vi "Intake_Joint_Execute.vi"() -> ()   [LabVIEW 2018]
uses:
  <vilib>/Rock Robotics/WPI/DriverStation/WPI_DriverStationRobotMode2.ctl
  <vilib>/Rock Robotics/WPI/ThirdParty/Phoenix-LabVIEW/Motor Controller/Controls/CTRE_Phoenix_MotorControl_ControlMode.ctl
  Global_Variables/Intake_Joint_Globals.vi
  Global_Variables/Sensor_Values.vi
  Global_Variables/Robot_Global_Data.vi
  Global_Variables/Dashboard_Globals.vi
panel:
  in  "Current_Position":dbl
  in  "Max_Speed":dbl=0.75 format="%#_13g"
  in  "Gain_Down":dbl=0.00025
  in  "Gain_Up":dbl=0.0006
  in  "Decrement":dbl=60.0
  in  "Increment":dbl=60.0
  in  "Gain":dbl=0.0009
  in  "Down_Speed":dbl=-0.3
  in  "Up_Speed":dbl=0.35
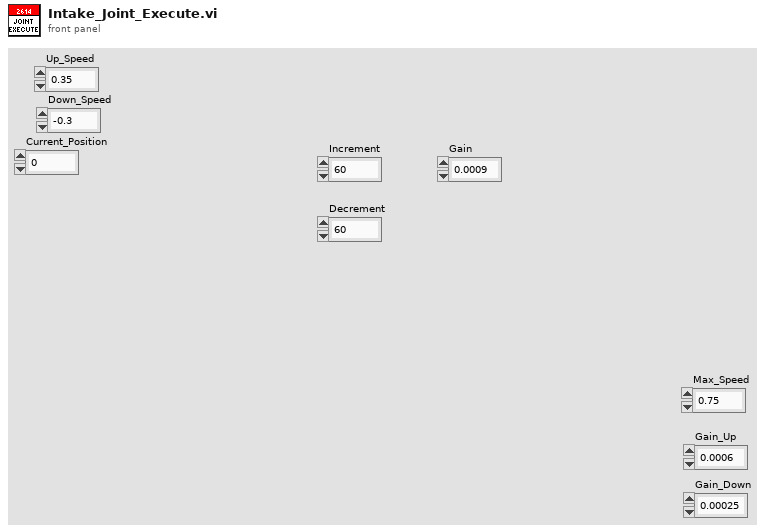
[diagram p1: front panel]
types:
  T1 = typedef "WPI_MotorControlDeviceRef.ctl" = cluster{"DeviceStatus":errorcluster, "Type":T2, "PWM":cluster{"PWM Channel":T3, "DeadBand":T4}, "CAN":cluster{"Device Number":u8, "SetOutput VI Ref":variant, "GetOutput VI Ref":variant, "Enable VI Ref":variant, "Disable VI Ref":variant, "Data":variant}, "Invert":bool, "DIO PWM":cluster{"PWM \"Enable\" Channel":T3, "DIOChannel":T5, "PWM Rate":dbl}}
  T2 = typedef "WPI_MotorControlType.ctl" = enum16{"PWM", "CAN", "DIO PWM"}
  T3 = typedef "FPGA_DIOPWMChannel.ctl" = enum8{"PWM 0", "PWM 1", "PWM 2", "PWM 3", "PWM 4", "PWM 5", "PWM 6", "PWM 7", "PWM 8", "PWM 9", "PWM MXP 0", "PWM MXP 1", "PWM MXP 2", "PWM MXP 3", "PWM MXP 4", "PWM MXP 5", "PWM MXP 6", "PWM MXP 7", "PWM MXP 8", "PWM MXP 9", "Invalid"}
  T4 = typedef "WPI_PWMDeadband.ctl" = cluster{"Name":string, "maxPositivePwm":i32, "minPositivePwm":i32, "centerPwm":i32, "maxNegativePwm":i32, "minNegativePwm":i32, "angularRange":u16}
  T5 = typedef "FPGA_DIOChannel.ctl" = enum8{"DIO 0", "DIO 1", "DIO 2", "DIO 3", "DIO 4", "DIO 5", "DIO 6", "DIO 7", "DIO 8", "DIO 9", "DIO MXP 0", "DIO MXP 1", "DIO MXP 2", "DIO MXP 3", "DIO MXP 4", "DIO MXP 5", "DIO MXP 6", "DIO MXP 7", "DIO MXP 8", "DIO MXP 9", "DIO MXP 10", "DIO MXP 11", "DIO MXP 12", "DIO MXP 13", "DIO MXP 14", "DIO MXP 15", "SPI Port CS1", "SPI Port CS2", "SPI Port CS3", "SPI Port MISO", "SPI Port MOSI", "Invalid"}
  T6 = typedef "WPI_DriverStationRobotMode2.ctl" = enum16{"Autonomous Disabled", "Autonomous Enabled", "Teleop Disabled", "Teleop Enabled", "Disconnected", "Finish", "Test Disabled", "Test Enabled", "Emergency Stopped"}
  T7 = typedef "Intake_Joint_Notifier.ctl" = cluster{"Intake_Joint_Control_Type":T8, "Manual_Joint_Up":bool, "Manual_Joint_Down":bool, "Low_Rocket":bool, "Mid_Rocket":bool, "High_Rocket":bool, "Cargo_Ship":bool, "Hatch_Floor":bool, "Cargo_Floor":bool, "HP_Hatch":bool, "HP_Cargo":bool, "Depot_Cargo":bool, "Stow":bool, "Intake_Mode":bool, "Set Position":T9, "Parameter_One":dbl, "Parameter_Two":dbl, "Parameter_Three":dbl, "Step":i32, "Joint_Notifier":refnum<notifier>}
  T8 = typedef "Intake_Joint_Control_Type.ctl" = enum16{"No_Op", "Manual_Joint_Up", "Manual_Joint_Down", "Manual_Position_Control", "Position_Control", "Position"}
  T9 = typedef "Intake_Joint_Enum_States.ctl" = enum16{"Current_Position", "High_Rocket_Hatch_Panel_Floor", "High_Rocket_Hatch_Panel", "Mid_Rocket_Hatch_Panel_Floor", "Mid_Rocket_Hatch_Panel", "Low_Rocket_Hatch_Panel", "Cargo_Ship_Hatch_Panel", "Loading_Station_Hatch_Panel", "Ground_Pickup_Hatch_Panel", "High_Rocket_Cargo", "Mid_Rocket_Cargo", "Low_Rocket_Cargo", "Cargo_Ship_Cargo", "Loading_Station_Cargo", "Ground_Pickup_Cargo", "Depot_Pickup_Cargo", "Stow_Cargo", "Get_Hatch"}
  T10 = typedef "CTRE_Phoenix_MotorControl_ControlMode.ctl" = u16
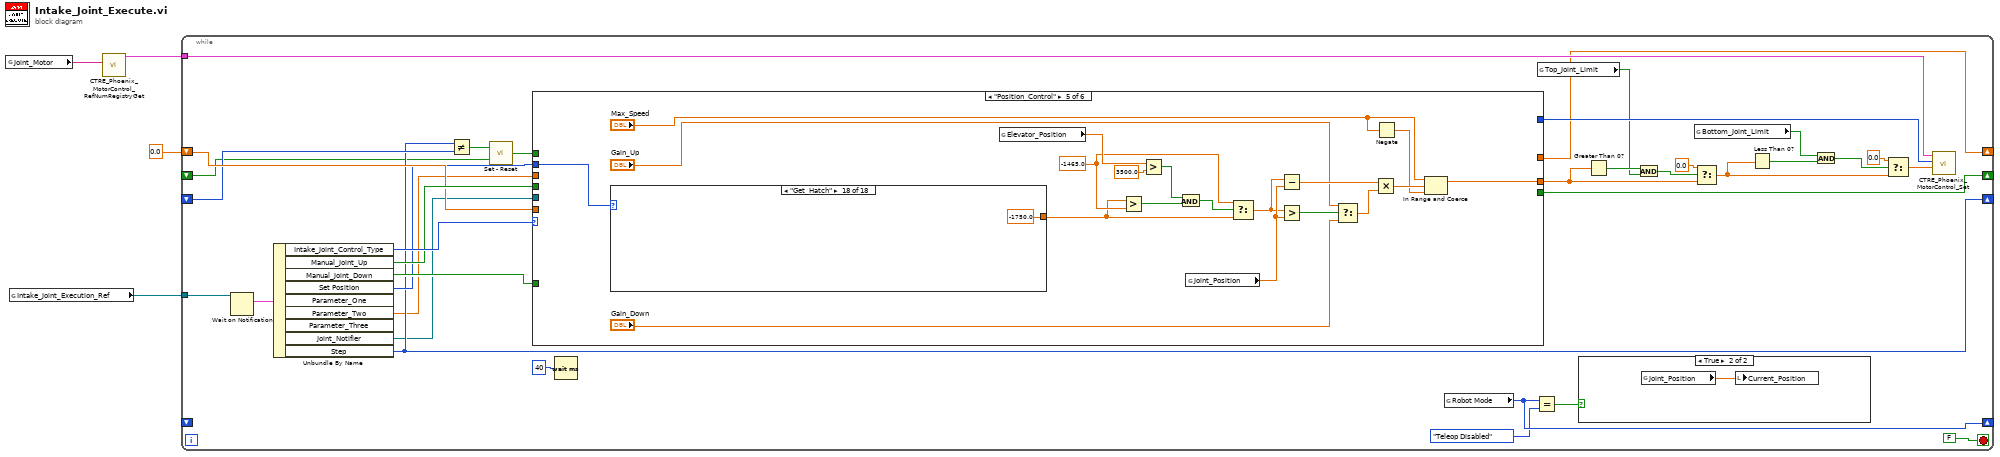
[diagram p0: block diagram]
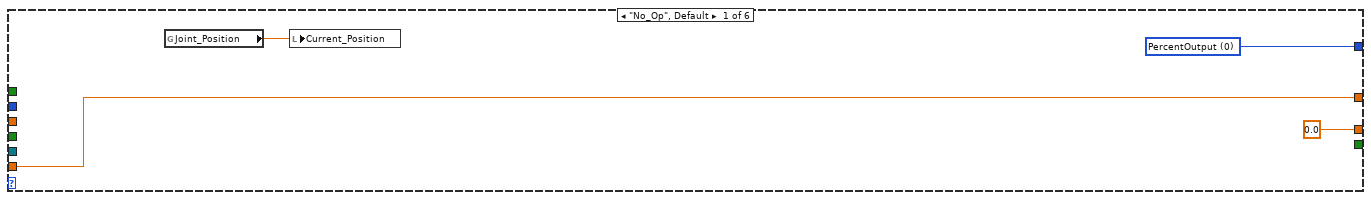
[diagram p3: hidden frame]
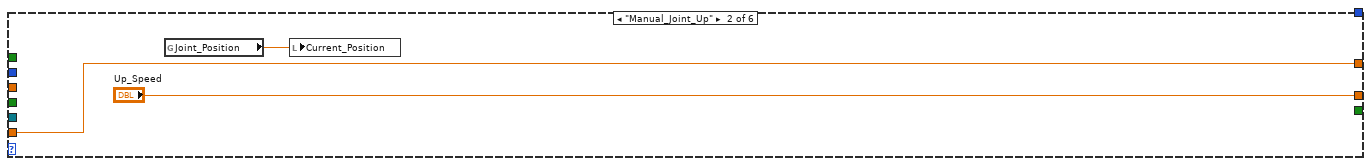
[diagram p4: hidden frame]
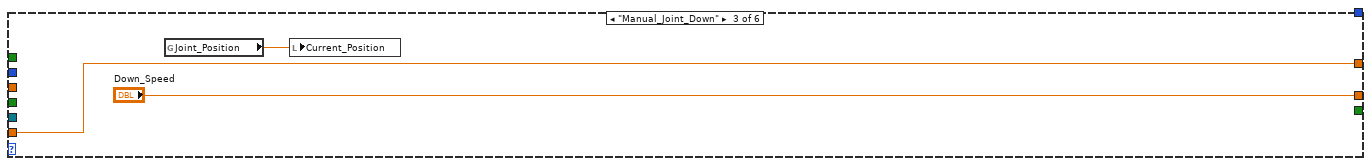
[diagram p5: hidden frame]
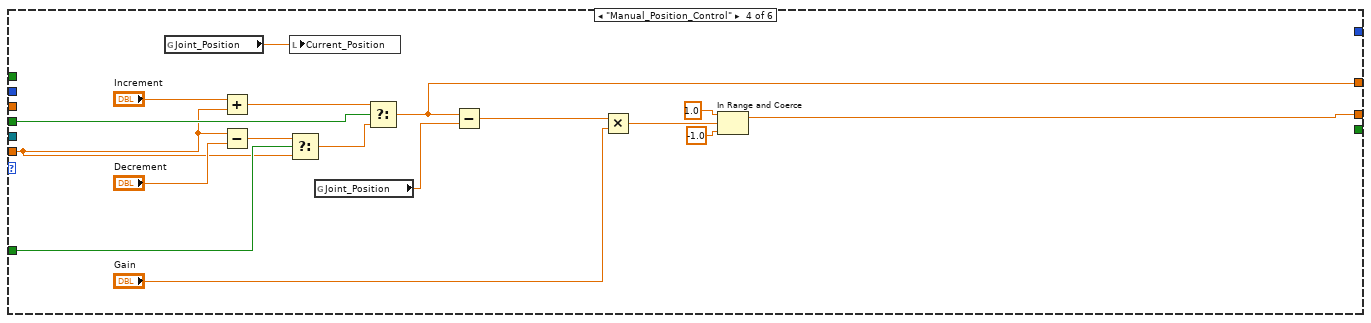
[diagram p6: hidden frame]
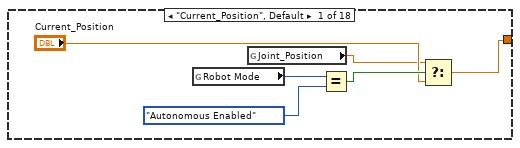
[diagram p7: hidden frame]
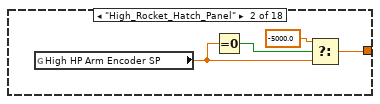
[diagram p8: hidden frame]
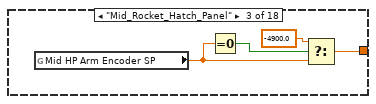
[diagram p9: hidden frame]
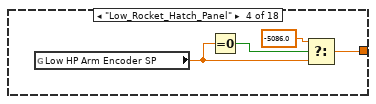
[diagram p10: hidden frame]
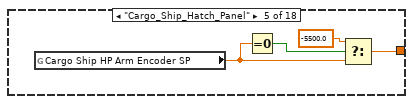
[diagram p11: hidden frame]
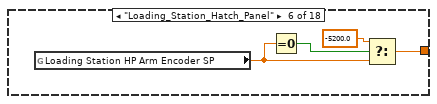
[diagram p12: hidden frame]
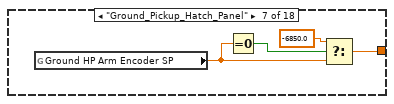
[diagram p13: hidden frame]
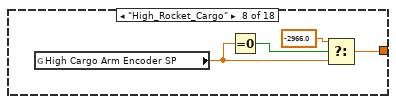
[diagram p14: hidden frame]
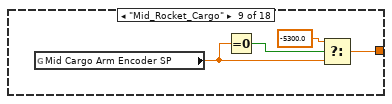
[diagram p15: hidden frame]
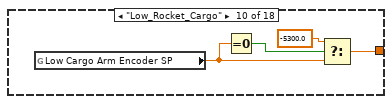
[diagram p16: hidden frame]
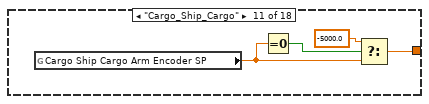
[diagram p17: hidden frame]
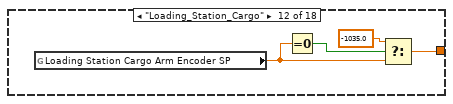
[diagram p18: hidden frame]
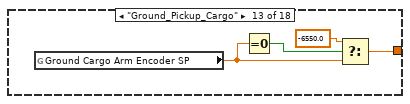
[diagram p19: hidden frame]
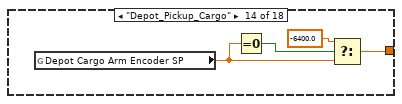
[diagram p20: hidden frame]
diagram:
  n1 = global read "Intake_Joint_Globals.vi" "Joint_Motor"() -> (w2:string)
  n2 = global read "Intake_Joint_Globals.vi" "Intake_Joint_Execution_Ref"() -> (w3:refnum<notifier>)
  n3 = call <vilib>:"CTRE_Phoenix_MotorControl_RefNumRegistryGet.vi"("refnum name"=w2) -> ("PhoenixMotorControlDevRef"=w4:T1)  [unwired: 9 in, 1 out]
  n4 = while {
    tunnel: w4 -> [w34]
    tunnel: w3 -> [w32]
    shift-right: [w17] -> _
    shift-left: 0.0 -> [w18]
    shift-right: [w13] -> _
    shift-left: _ -> [w11]
    shift-right: [w14] -> _
    shift-left: _ -> [w15]
    shift-right: [w7] -> _
    shift-left: _ -> [_]
    stop <- FALSE stop-if-true
    n5 = Wait on Notification(notifier=w32) -> (notification=w36:T7)  [unwired: 3 in, 3 out]
    n6 = Unbundle By Name(w36) -> ("Intake_Joint_Control_Type"=w35:T8, "Manual_Joint_Up"=w19:bool, "Manual_Joint_Down"=w20:bool, "Set Position"=w16:T9, "Parameter_Two"=w9:dbl, "Joint_Notifier"=w8:refnum<notifier>, "Step"=w14:i32)  [unwired: 2 out]
    n7 = Not Equal?(x=w14, y=w15) -> (x != y?=w12:bool)
    n8 = call "Set - Reset.vi"("Reset"=w11, "Set"=w12) -> ("Output"=w10:bool)
    n9 = case shown="\"Position_Control\"" w35 {
      tunnel: [w43 _ _ _ _ _] -> w33
      tunnel: [0.0 ("Output") "Up_Speed" "Down_Speed" w63 w78 w158] -> w22
      tunnel: w20 -> [_ _ _ w56 _ _]
      tunnel: w19 -> [_ _ _ w60 _ _]
      tunnel: w18 -> [w41 w45 w48 w53 _ w163]
      tunnel: [w41 w45 w48 w52 _ _] -> w17
      tunnel: w16 -> [_ _ _ _ w75 w161]
      tunnel: [_ _ _ _ _ w165] -> w13
      tunnel: w10 -> [_ _ _ _ _ w164]
      tunnel: w9 -> [_ _ _ _ _ w162]
      tunnel: w8 -> [_ _ _ _ _ w159]
      frame "No_Op", Default {
        w43 = T10 0 items=["PercentOutput"=0, "Position"=1, "Velocity"=2, "Current"=3, "Follower"=5, "MotionProfile"=6, "MotionMagic"=7, "MotionProfileArc"=10, "Disabled"=15] ("Control Mode")
        n10 = global read "Sensor_Values.vi" "Joint_Position"() -> (w40:dbl)
        n11 = local write "Current_Position"(w40) -> ()
      }
      frame "Manual_Joint_Up" {
        n12 = global read "Sensor_Values.vi" "Joint_Position"() -> (w44:dbl)
        n13 = local write "Current_Position"(w44) -> ()
      }
      frame "Manual_Joint_Down" {
        n14 = global read "Sensor_Values.vi" "Joint_Position"() -> (w47:dbl)
        n15 = local write "Current_Position"(w47) -> ()
      }
      frame "Manual_Position_Control" {
        n16 = global read "Sensor_Values.vi" "Joint_Position"() -> (w50:dbl)
        n17 = Add(x="Increment", y=w53) -> (x+y=w59:dbl)
        n18 = Subtract(x=w53, y="Decrement") -> (x-y=w55:dbl)
        n19 = local write "Current_Position"(w50) -> ()
        n20 = Select(t=w55, s=w56, f=w53) -> (s? t:f=w57:dbl)
        n21 = global read "Sensor_Values.vi" "Joint_Position"() -> (w51:dbl)
        n22 = Select(t=w59, s=w60, f=w57) -> (s? t:f=w52:dbl)
        n23 = Subtract(x=w52, y=w51) -> (x-y=w66:dbl)
        n24 = Multiply(x=w66, y="Gain") -> (x*y=w64:dbl)
        n25 = In Range and Coerce(upper limit=1.0, x=w64, lower limit=-1.0) -> (coerced(x)=w63:dbl)  [unwired: 1 out]
      }
      frame "Position_Control" {
        w69 = -1465.0 ("y")
        n26 = case shown="\"Get_Hatch\"" w75 {
          tunnel: [w87 w92 w97 w101 w105 w109 w113 w117 w121 w125 w128 w133 w137 w140 w145 w149 w153 -1750.0 ("Mid HP Floor Arm Encoder SP")] -> w68
          frame "Current_Position", Default {
            n27 = global read "Robot_Global_Data.vi" "Robot Mode"() -> (w90:T6)
            n28 = global read "Sensor_Values.vi" "Joint_Position"() -> (w86:dbl)
            n29 = Equal?(x=w90, y=WPI_DriverStationRobotMode2."Autonomous Enabled") -> (x = y?=w89:bool)
            n30 = Select(t=w86, s=w89, f="Current_Position") -> (s? t:f=w87:dbl)
          }
          frame "High_Rocket_Hatch_Panel" {
            n31 = global read "Dashboard_Globals.vi" "High HP Arm Encoder SP"() -> (w93:dbl)
            n32 = Equal To 0?(x=w93) -> (x = 0?=w95:bool)
            n33 = Select(t=-5000.0, s=w95, f=w93) -> (s? t:f=w92:dbl)
          }
          frame "Mid_Rocket_Hatch_Panel" {
            n34 = global read "Dashboard_Globals.vi" "Mid HP Arm Encoder SP"() -> (w96:dbl)
            n35 = Equal To 0?(x=w96) -> (x = 0?=w99:bool)
            n36 = Select(t=-4900.0, s=w99, f=w96) -> (s? t:f=w97:dbl)
          }
          frame "Low_Rocket_Hatch_Panel" {
            n37 = global read "Dashboard_Globals.vi" "Low HP Arm Encoder SP"() -> (w100:dbl)
            n38 = Equal To 0?(x=w100) -> (x = 0?=w103:bool)
            n39 = Select(t=-5086.0, s=w103, f=w100) -> (s? t:f=w101:dbl)
          }
          frame "Cargo_Ship_Hatch_Panel" {
            n40 = global read "Dashboard_Globals.vi" "Cargo Ship HP Arm Encoder SP"() -> (w104:dbl)
            n41 = Equal To 0?(x=w104) -> (x = 0?=w107:bool)
            n42 = Select(t=-5500.0, s=w107, f=w104) -> (s? t:f=w105:dbl)
          }
          frame "Loading_Station_Hatch_Panel" {
            n43 = global read "Dashboard_Globals.vi" "Loading Station HP Arm Encoder SP"() -> (w108:dbl)
            n44 = Equal To 0?(x=w108) -> (x = 0?=w111:bool)
            n45 = Select(t=-5200.0, s=w111, f=w108) -> (s? t:f=w109:dbl)
          }
          frame "Ground_Pickup_Hatch_Panel" {
            n46 = global read "Dashboard_Globals.vi" "Ground HP Arm Encoder SP"() -> (w112:dbl)
            n47 = Equal To 0?(x=w112) -> (x = 0?=w115:bool)
            n48 = Select(t=-6850.0, s=w115, f=w112) -> (s? t:f=w113:dbl)
          }
          frame "High_Rocket_Cargo" {
            n49 = global read "Dashboard_Globals.vi" "High Cargo Arm Encoder SP"() -> (w116:dbl)
            n50 = Equal To 0?(x=w116) -> (x = 0?=w119:bool)
            n51 = Select(t=-2966.0, s=w119, f=w116) -> (s? t:f=w117:dbl)
          }
          frame "Mid_Rocket_Cargo" {
            n52 = global read "Dashboard_Globals.vi" "Mid Cargo Arm Encoder SP"() -> (w120:dbl)
            n53 = Equal To 0?(x=w120) -> (x = 0?=w123:bool)
            n54 = Select(t=-5300.0, s=w123, f=w120) -> (s? t:f=w121:dbl)
          }
          frame "Low_Rocket_Cargo" {
            n55 = global read "Dashboard_Globals.vi" "Low Cargo Arm Encoder SP"() -> (w124:dbl)
            n56 = Equal To 0?(x=w124) -> (x = 0?=w127:bool)
            n57 = Select(t=-5300.0, s=w127, f=w124) -> (s? t:f=w125:dbl)
          }
          frame "Cargo_Ship_Cargo" {
            n58 = global read "Dashboard_Globals.vi" "Cargo Ship Cargo Arm Encoder SP"() -> (w129:dbl)
            n59 = Equal To 0?(x=w129) -> (x = 0?=w131:bool)
            n60 = Select(t=-5000.0, s=w131, f=w129) -> (s? t:f=w128:dbl)
          }
          frame "Loading_Station_Cargo" {
            n61 = global read "Dashboard_Globals.vi" "Loading Station Cargo Arm Encoder SP"() -> (w132:dbl)
            n62 = Equal To 0?(x=w132) -> (x = 0?=w135:bool)
            n63 = Select(t=-1035.0, s=w135, f=w132) -> (s? t:f=w133:dbl)
          }
          frame "Ground_Pickup_Cargo" {
            n64 = global read "Dashboard_Globals.vi" "Ground Cargo Arm Encoder SP"() -> (w136:dbl)
            n65 = Equal To 0?(x=w136) -> (x = 0?=w139:bool)
            n66 = Select(t=-6550.0, s=w139, f=w136) -> (s? t:f=w137:dbl)
          }
          frame "Depot_Pickup_Cargo" {
            n67 = global read "Dashboard_Globals.vi" "Depot Cargo Arm Encoder SP"() -> (w141:dbl)
            n68 = Equal To 0?(x=w141) -> (x = 0?=w143:bool)
            n69 = Select(t=-6400.0, s=w143, f=w141) -> (s? t:f=w140:dbl)
          }
          frame "Stow_Cargo" {
            n70 = global read "Dashboard_Globals.vi" "Stow Cargo Arm Encoder SP"() -> (w144:dbl)
            n71 = Equal To 0?(x=w144) -> (x = 0?=w147:bool)
            n72 = Select(t=0.0, s=w147, f=w144) -> (s? t:f=w145:dbl)
          }
          frame "High_Rocket_Hatch_Panel_Floor" {
            n73 = global read "Dashboard_Globals.vi" "High HP Floor Arm Encoder SP"() -> (w148:dbl)
            n74 = Equal To 0?(x=w148) -> (x = 0?=w151:bool)
            n75 = Select(t=-2200.0, s=w151, f=w148) -> (s? t:f=w149:dbl)
          }
          frame "Mid_Rocket_Hatch_Panel_Floor" {
            n76 = global read "Dashboard_Globals.vi" "Mid HP Floor Arm Encoder SP"() -> (w152:dbl)
            n77 = Equal To 0?(x=w152) -> (x = 0?=w155:bool)
            n78 = Select(t=-1470.0, s=w155, f=w152) -> (s? t:f=w153:dbl)
          }
          frame "Get_Hatch" {
          }
        }
        n79 = global read "Sensor_Values.vi" "Elevator_Position"() -> (w74:dbl)
        n80 = Greater?(x=w68, y=w69) -> (0:w71:bool)
        n81 = Greater?(x=w74, y=3500.0) -> (0:w72:bool)
        n82 = And(x=w72, y=w71) -> (x .and. y?=w70:bool)
        n83 = global read "Sensor_Values.vi" "Joint_Position"() -> (w76:dbl)
        n84 = Select(t=w69, s=w70, f=w68) -> (s? t:f=w67:dbl)
        n85 = Subtract(x=w67, y=w76) -> (x-y=w85:dbl)
        n86 = Greater?(x=w67, y=w76) -> (0:w77:bool)
        n87 = Select(t="Gain_Up", s=w77, f="Gain_Down") -> (s? t:f=w82:dbl)
        n88 = Multiply(x=w85, y=w82) -> (x*y=w81:dbl)
        n89 = Negate(x="Max_Speed") -> (-x=w79:dbl)
        n90 = In Range and Coerce(upper limit="Max_Speed", x=w81, lower limit=w79) -> (coerced(x)=w78:dbl)  [unwired: 1 out]
      }
      frame "Position" {
        n91 = call "Command_Arm.vi"("Timeout"=w162, "Allowable_Error"=w163, "Set Position"=w161, "Startup"=w164) -> ("Reinit"=w165:bool, "Motor_Out"=w158:dbl, "Completed"=w160:bool)
        n92 = global read "Sensor_Values.vi" "Joint_Position"() -> (w157:dbl)
        n93 = Send Notification(notification=w160, notifier=w159) -> ()  [unwired: 1 in, 2 out]
        n94 = local write "Current_Position"(w157) -> ()
      }
    }
    n95 = Wait (ms)(milliseconds to wait=u32 40) -> ()  [unwired: 1 out]
    n96 = global read "Robot_Global_Data.vi" "Robot Mode"() -> (w7:T6)
    n97 = Equal?(x=w7, y=WPI_DriverStationRobotMode2."Teleop Disabled") -> (x = y?=w5:bool)
    n98 = global read "Sensor_Values.vi" "Top_Joint_Limit"() -> (w30:bool)
    n99 = case shown="True" w5 {
      frame False {
      }
      frame True {
        n100 = global read "Sensor_Values.vi" "Joint_Position"() -> (w39:dbl)
        n101 = local write "Current_Position"(w39) -> ()
      }
    }
    n102 = Greater Than 0?(x=w22) -> (x > 0?=w31:bool)
    n103 = And(x=w31, y=w30) -> (x .and. y?=w29:bool)
    n104 = global read "Sensor_Values.vi" "Bottom_Joint_Limit"() -> (w25:bool)
    n105 = Select(t=0.0, s=w29, f=w22) -> (s? t:f=w23:dbl)
    n106 = Less Than 0?(x=w23) -> (x < 0?=w24:bool)
    n107 = And(x=w25, y=w24) -> (x .and. y?=w26:bool)
    n108 = Select(t=0.0, s=w26, f=w23) -> (s? t:f=w21:dbl)
    n109 = call <vilib>:"CTRE_Phoenix_MotorControl_Set.vi"("Output"=w21, "Control Mode"=w33, "PhoenixMotorControlDevRef"=w34) -> ()  [unwired: 7 in, 2 out]
  }
